vi "IPC-Modbus-Transfer-DecodeRequest-WriteMulRegisters.vi"(4 "无符号字节数组":u8[](array[numeric])) -> (1 "Write Multiple Registers request":T1)   [LabVIEW 2014]
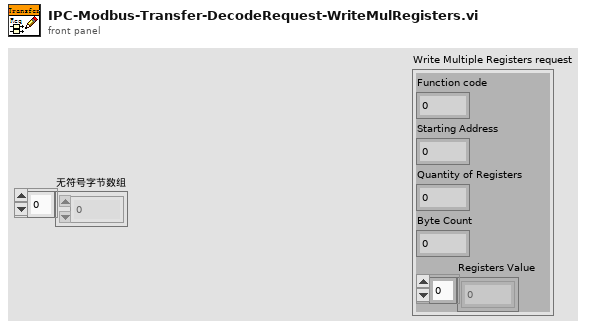
[diagram p1: front panel]
types:
  T1 = cluster{"Function code":u8, "Starting Address":u16, "Quantity of Registers":u16, "Byte Count":u8, "Registers Value":u16[]}
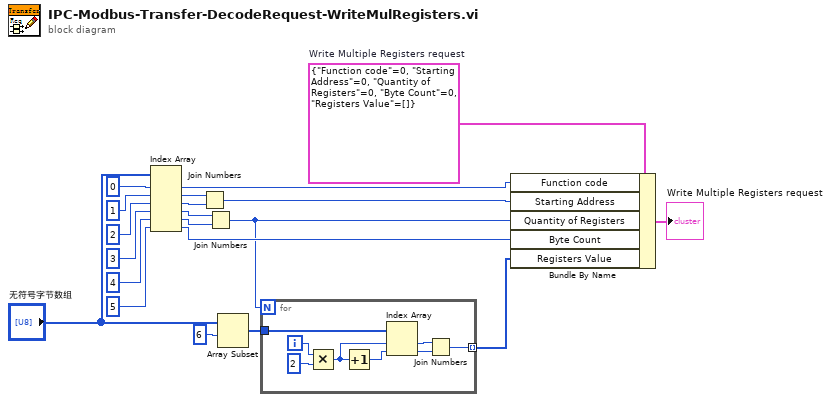
[diagram p0: block diagram]
diagram:
  w9 = T1 {"Function code"=0, "Starting Address"=0, "Quantity of Registers"=0, "Byte Count"=0, "Registers Value"=[]}  # Write Multiple Registers request
  n1 = Index Array(array="无符号字节数组", index #1=0 ("索引"), index #2=1 ("索引"), index #3=2 ("索引"), index #4=3 ("索引"), index #5=4 ("索引"), index #6=5 ("索引")) -> (element #1=w15:u8, element #2=w14:u8, element #3=w13:u8, element #4=w11:u8, element #5=w10:u8, element #6=w8:u8)
  n2 = Join Numbers(hi=w14, lo=w13) -> ((hi.lo)=w12:u16)
  n3 = Join Numbers(hi=w11, lo=w10) -> ((hi.lo)=w6:u16)
  n4 = Array Subset(array="无符号字节数组", index=6 ("索引")) -> (w3:u8[])  [unwired: 1 in]
  n5 = for {
    N: w6 -> [_]
    tunnel: w3 -> [w28]
    tunnel: [w21] -> w2 mode=indexing
    i -> [w27]
    n6 = Multiply(x=w27, y=2) -> (x*y=w25:i32)
    n7 = Increment(x=w25) -> (x+1=w24:i32)
    n8 = Index Array(array=w28, index #1=w25, index #2=w24) -> (element #1=w23:u8, element #2=w22:u8)
    n9 = Join Numbers(hi=w23, lo=w22) -> ((hi.lo)=w21:u16)
  }
  n10 = Bundle By Name(cluster=w9, "Function code"=w15, "Starting Address"=w12, "Quantity of Registers"=w6, "Byte Count"=w8, "Registers Value"=w2) -> (→"Write Multiple Registers request":T1)
